vi "SaveLoadPrev-section.vi"(3 "file path (use dialog)":path=path "F:/control db/control software/Control vi/Temp control/ion Source Test.txt", 4 "Cluster 2":T1, 5 "VI Refnum":refnum<vi>) -> (0 "error out":errorcluster)   [LabVIEW 2016, in "SaveLoad.lvlib"]
doc: "This vi allows a section to save or load a control settings file to/from disk"
uses:
  SaveLoad.lvlib
  saveloadprev.ctl
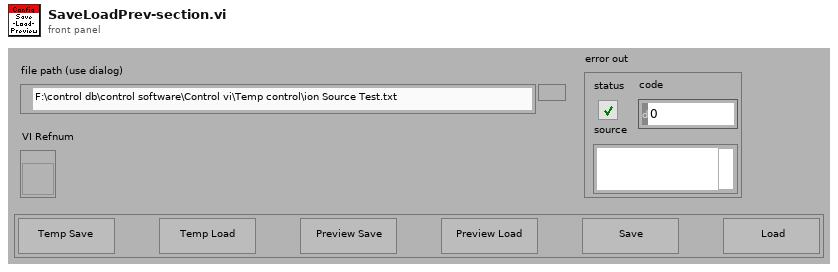
[diagram p1: front panel]
types:
  T1 = typedef "saveloadprev.ctl" = cluster{"Temp Save":bool, "Temp Load":bool, "Save":bool, "Load":bool, "Preview Save":bool, "Preview Load":bool}
  T2 = typedef "prev-save-load-enum.ctl" = enum16{"Temp Save", "Temp Load", "Save", "Load", "Preview Save", "Preview Load"}
  T3 = enum16{"open", "replace", "create", "open or create", "replace or create", "replace or create with confirmation"}
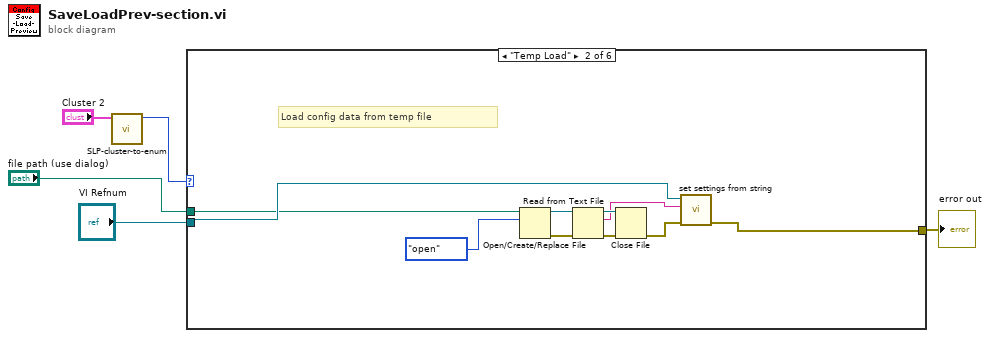
[diagram p0: block diagram]
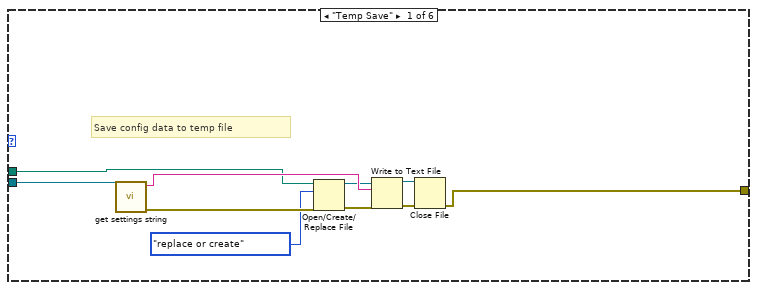
[diagram p2: hidden frame]
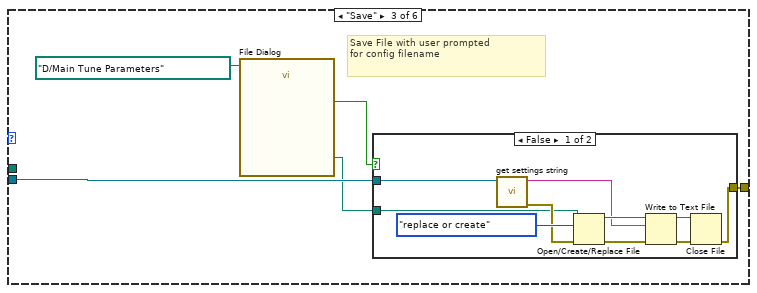
[diagram p3: hidden frame]
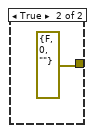
[diagram p4: hidden frame]
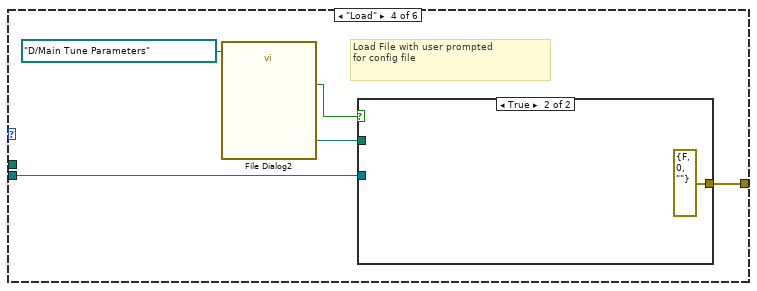
[diagram p5: hidden frame]
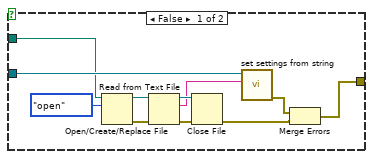
[diagram p6: hidden frame]
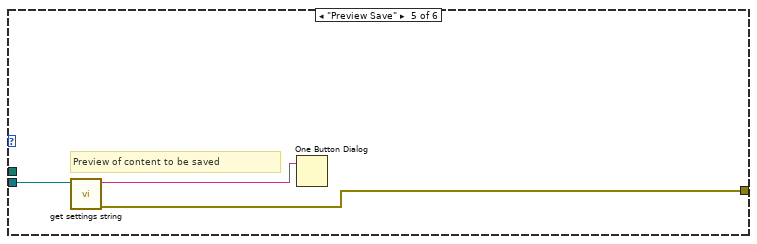
[diagram p7: hidden frame]
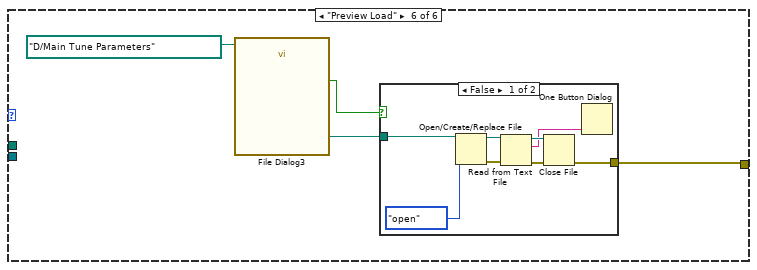
[diagram p8: hidden frame]
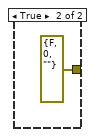
[diagram p9: hidden frame]
diagram:
  n1 = call "SLP-cluster-to-enum.vi"("Prev-Save-Load"="Cluster 2") -> ("Prev-Save-Load enum"=w1:T2)  [unwired: 10 in]
  n2 = case shown="\"Temp Load\"" w1 {
    tunnel: "VI Refnum" -> [w13 w20 w30 w45 w61 _]
    tunnel: "file path (use dialog)" -> [w8 w18 _ _ _ _]
    tunnel: [w11 w21 w29 w46 w59 w65] -> w4
    frame "Temp Save" {
      # "Save config data to temp file"
      n3 = call "get settings string.vi"("VI in"=w13) -> ("error out"=w10:errorcluster, "Settings string"=w12:string)  [unwired: 9 in]
      n4 = Open/Create/Replace File(file path (use dialog)=w8, error in=w10, operation (0:open)=T3."replace or create") -> (refnum out=w7:refnum<file>, error out=w9:errorcluster)  [unwired: 3 in, 1 out]
      n5 = Write to Text File(file (use dialog)=w7, text=w12, error in=w9) -> (refnum out=w15:refnum<file>, error out=w14:errorcluster)  [unwired: 1 in, 1 out]
      n6 = Close File(refnum=w15, error in=w14) -> (error out=w11:errorcluster)  [unwired: 1 out]
    }
    frame "Temp Load" {
      # "Load config data from temp file"
      n7 = Open/Create/Replace File(file path (use dialog)=w18, operation (0:open)=T3."open") -> (refnum out=w17:refnum<file>, error out=w19:errorcluster)  [unwired: 4 in, 1 out]
      n8 = Read from Text File(file (use dialog)=w17, error in=w19) -> (refnum out=w25:refnum<file>, text=w23:string, error out=w24:errorcluster)  [unwired: 3 out]
      n9 = Close File(refnum=w25, error in=w24) -> (error out=w22:errorcluster)  [unwired: 1 out]
      n10 = call "set settings from string.vi"("error constant"=w22, "String"=w23, "VI in"=w20) -> ("error out"=w21:errorcluster)  [unwired: 8 in]
    }
    frame "Save" {
      # "Save File with user prompted\nfor config filename"
      n11 = call "File Dialog"("start path"=path "D:/Main Tune Parameters") -> ("selected path"=w27:path, "cancelled"=w26:bool)  [unwired: 11 in, 2 out]
      n12 = case shown="False" w26 {
        tunnel: w30 -> [w35 _]
        tunnel: [w32 errorcluster {"status"=FALSE, "code"=0, "source"=""} ("error out")] -> w29
        tunnel: w27 -> [w31 _]
        frame False {
          n13 = call "get settings string.vi"("VI in"=w35) -> ("error out"=w33:errorcluster, "Settings string"=w34:string)  [unwired: 9 in]
          n14 = Open/Create/Replace File(file path (use dialog)=w31, error in=w33, operation (0:open)=T3."replace or create") -> (refnum out=w38:refnum<file>, error out=w37:errorcluster)  [unwired: 1 in, 3 out]
          n15 = Write to Text File(file (use dialog)=w38, text=w34, error in=w37) -> (refnum out=w39:refnum<file>, error out=w40:errorcluster)  [unwired: 1 in, 1 out]
          n16 = Close File(refnum=w39, error in=w40) -> (error out=w32:errorcluster)  [unwired: 1 out]
        }
        frame True {
        }
      }
    }
    frame "Load" {
      # "Load File with user prompted\nfor config file"
      n17 = call "File Dialog2"("start path"=path "D:/Main Tune Parameters") -> ("selected path"=w44:path, "cancelled"=w42:bool)  [unwired: 11 in, 2 out]
      n18 = case shown="True" w42 {
        tunnel: [w53 errorcluster {"status"=FALSE, "code"=0, "source"=""} ("error IO")] -> w46
        tunnel: w45 -> [w51 _]
        tunnel: w44 -> [w48 _]
        frame False {
          n19 = Open/Create/Replace File(file path (use dialog)=w48, operation (0:open)=T3."open") -> (refnum out=w49:refnum<file>, error out=w50:errorcluster)  [unwired: 2 in, 3 out]
          n20 = Read from Text File(file (use dialog)=w49, error in=w50) -> (refnum out=w56:refnum<file>, text=w55:string, error out=w57:errorcluster)  [unwired: 3 out]
          n21 = Close File(refnum=w56, error in=w57) -> (error out=w54:errorcluster)  [unwired: 1 out]
          n22 = call "set settings from string.vi"("String"=w55, "VI in"=w51) -> ("error out"=w52:errorcluster)  [unwired: 9 in]
          n23 = Merge Errors(w52, w54) -> (w53:errorcluster)
        }
        frame True {
        }
      }
    }
    frame "Preview Save" {
      # "Preview of content to be saved"
      n24 = call "get settings string.vi"("VI in"=w61) -> ("error out"=w59:errorcluster, "Settings string"=w60:string)  [unwired: 9 in]
      n25 = One Button Dialog(message=w60) -> ()  [unwired: 1 in, 1 out]
    }
    frame "Preview Load" {
      n26 = call "File Dialog3"("start path"=path "D:/Main Tune Parameters") -> ("selected path"=w63:path, "cancelled"=w62:bool)  [unwired: 11 in, 2 out]
      n27 = case shown="False" w62 {
        tunnel: [w70 errorcluster {"status"=FALSE, "code"=0, "source"=""} ("error out")] -> w65
        tunnel: w63 -> [w67 _]
        frame False {
          n28 = Open/Create/Replace File(file path (use dialog)=w67, operation (0:open)=T3."open") -> (refnum out=w68:refnum<file>, error out=w69:errorcluster)  [unwired: 4 in, 1 out]
          n29 = Read from Text File(file (use dialog)=w68, error in=w69) -> (refnum out=w73:refnum<file>, text=w72:string, error out=w71:errorcluster)  [unwired: 3 out]
          n30 = Close File(refnum=w73, error in=w71) -> (error out=w70:errorcluster)  [unwired: 1 out]
          n31 = One Button Dialog(message=w72) -> ()  [unwired: 1 in, 1 out]
        }
        frame True {
        }
      }
    }
  }
  "error out" <- w4
